vi "Create Relay Status Arrays.vi"(8 "error in":errorcluster, 11 "SwitchMatrix in":refnum<class "SwitchMatrix.lvclass">) -> (0 "error out":errorcluster, 3 "SwitchMatrix out":refnum<class "SwitchMatrix.lvclass">)   [LabVIEW 2019, in "SwitchMatrix.lvlib" / "SwitchMatrix.lvclass"]
doc: "Create arrays of both relay names and relay states. This reserves the memory block for these values. It is the child class developer's responsibility to read the relay names from the instrument and overwrite the empty string constants for the relay names."
uses:
  Library/SwitchMatrix.lvclass
  Library/SwitchMatrix.lvclass/SwitchMatrix.ctl
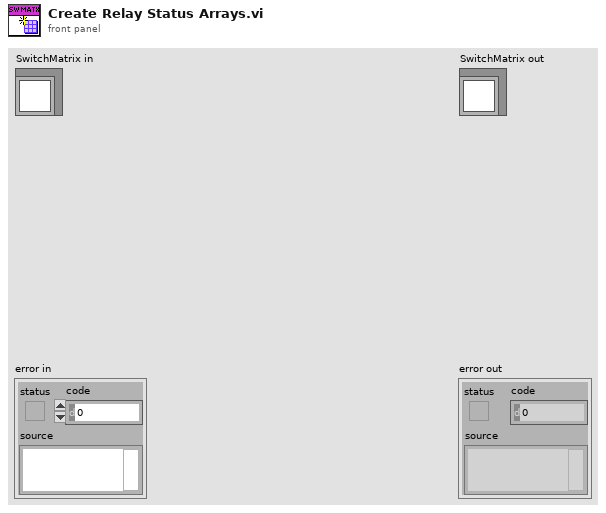
[diagram p1: front panel]
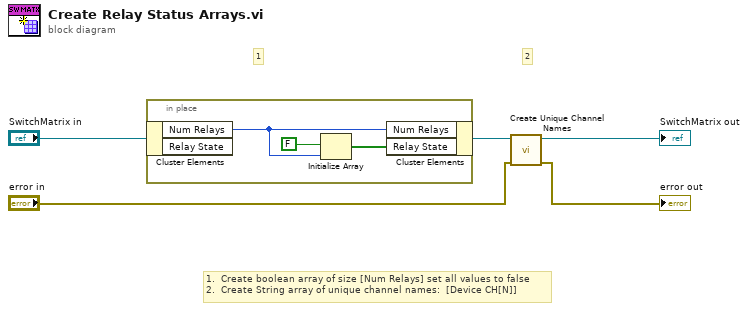
[diagram p0: block diagram]
diagram:
  # "1.  Create boolean array of size [Num Relays] set all values to false\n2.  Create String array of unique channel names:  [Device CH[N]]"
  # "2"
  # "1"
  n1 = in-place {
    # "Create memory space for [Num Relays] states."
    n2 = in-place-cluster #1("SwitchMatrix in") -> ("Num Relays"=w6:i32)  [unwired: 1 out]
    n3 = Initialize Array(FALSE, w6) -> (w7:bool[])
    n4 = in-place-cluster #1("Num Relays"=w6, "Relay State"=w7) -> (w4:refnum<class "SwitchMatrix.lvclass">)
  }
  n5 = call "Create Unique Channel Names.vi"("error in"="error in", "SwitchMatrix in"=w4) -> ("error out"=→"error out":errorcluster, "SwitchMatrix out"=→"SwitchMatrix out":refnum<class "SwitchMatrix.lvclass">)  [unwired: 8 in]
